vi "Auton Disabled Simulator.vi"() -> ()   [LabVIEW 2015]
panel:
  out "Value Sequence":dbl[][](array[numeric])
  out "Type Sequence":string[][](array[string])
  out "Auton Sequence":T1
  out "Selected Script":string
  in  "Down":bool
  in  "Up":bool
  in  "stop":bool
  out "Script Path":string
  out "filenames":string[](array[string])
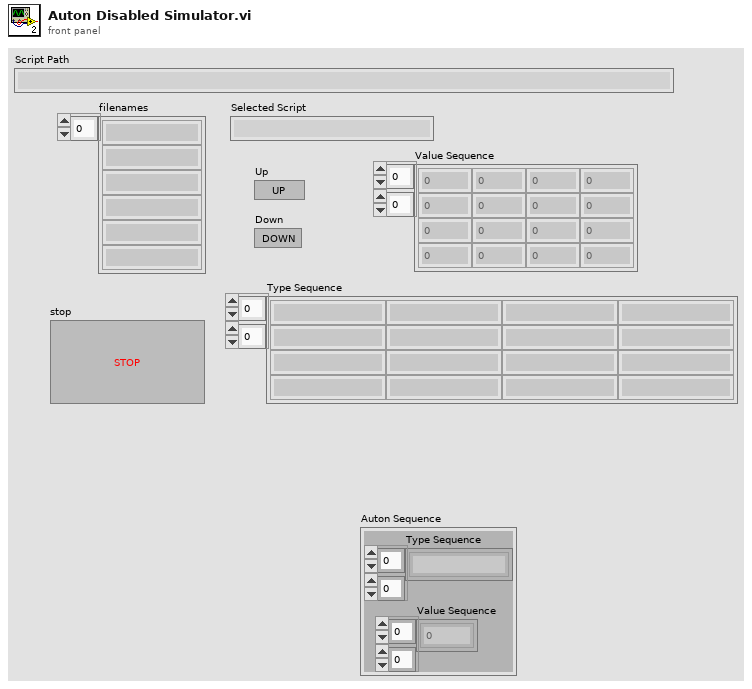
[diagram p1: front panel]
types:
  T1 = cluster{"Type Sequence":string[][], "Value Sequence":dbl[][]}
  T2 = cluster{"Paramter Type":string[], "Parameter Values":dbl[]}
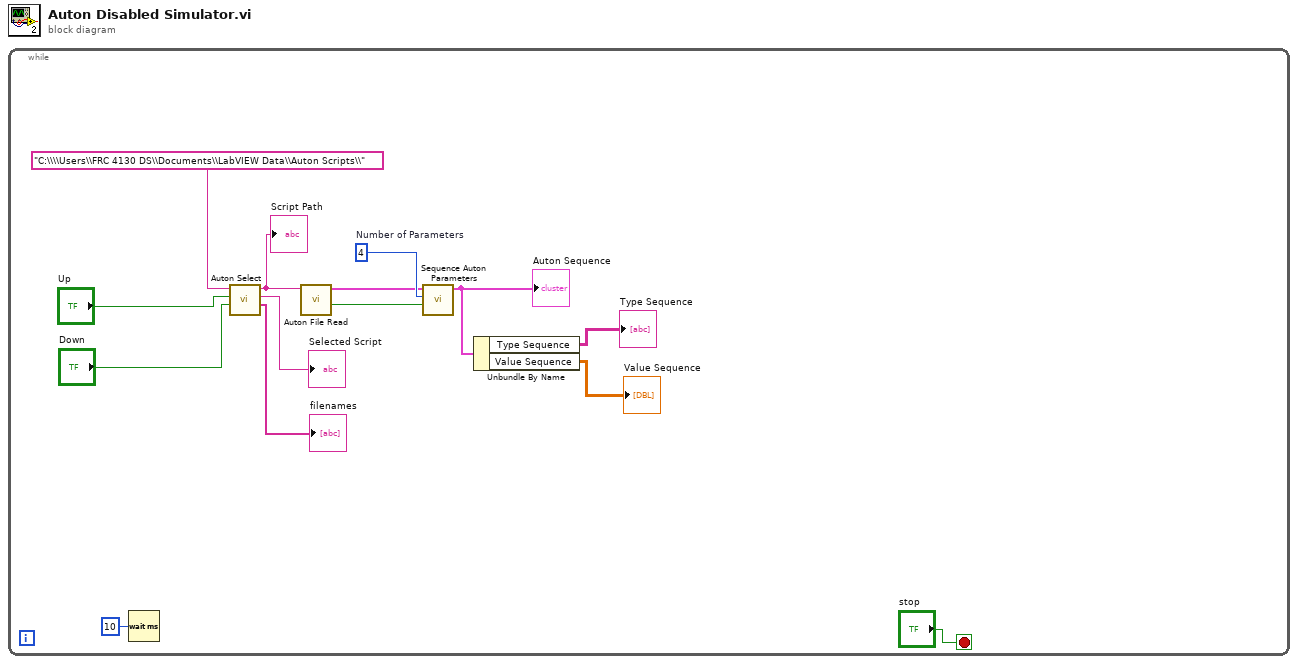
[diagram p0: block diagram]
diagram:
  n1 = while {
    stop <- "stop" stop-if-true
    w6 = 4  # Number of Parameters
    n2 = Wait (ms)(milliseconds to wait=u32 10) -> ()  [unwired: 1 out]
    n3 = call "Auton Select.vi"("Select Previous"="Down", "Select Next"="Up", "Script Folder Path"="C:\\\\Users\\FRC 4130 DS\\Documents\\LabVIEW Data\\Auton Scripts\\" ("string")) -> ("filenames"=→"filenames":string[], "Selected Script"=→"Selected Script":string, "Script Path"=w7:string)  [unwired: 5 in, 1 out]
    "Script Path" <- w7
    n4 = call "Auton File Read.vi"("Script Path"=w7) -> ("New Script Loaded"=w1:bool, "Auton Parameters"=w5:T2)  [unwired: 8 in, 1 out]
    n5 = call "Sequence Auton Parameters.vi"("Parse Parameters?"=w1, "Number of Parameters"=w6, "Auton Parameters"=w5) -> ("Auton Sequence"=w4:T1)  [unwired: 7 in, 1 out]
    "Auton Sequence" <- w4
    n6 = Unbundle By Name(w4) -> ("Type Sequence"=→"Type Sequence":string[][], "Value Sequence"=→"Value Sequence":dbl[][])
  }
